vi "Reset Sensors.vi"   [LabVIEW 2014]
uses:
  Elevator/Elevator Control Command.ctl
  Elevator/Elevator Command.ctl
  Common Code/Elevator Mode.ctl
  Robot Global Data.vi
types:
  T1 = typedef "Elevator Command.ctl" = enum16{"Idle", "Load 1", "Load 2", "Load 3", "Drop Stack", "Eject Stack", "Untip Trashcan", "Load Trashcan"}
  T2 = typedef "Elevator Mode.ctl" = enum16{"Manual", "Safe", "Auto"}
  T3 = typedef "Elevator Control Command.ctl" = cluster{"Command":T1, "Manual Motor Out":dbl, "Manual Eject Piston":bool, "Mode":T2, "Override Limits":bool, "Manual Stabilizer":bool, "Manual Finger":bool, "Load from Step?":bool, "Store Trashcan?":bool, "Hold Low?":bool}
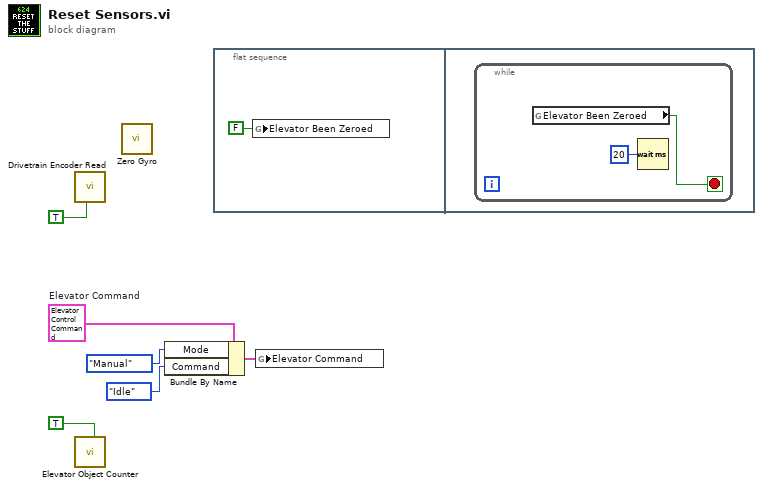
[diagram p0: block diagram]
diagram:
  w5 = T3 {"Command"=enum."Idle", "Manual Motor Out"=0.007874015748031496, "Manual Eject Piston"=FALSE, "Mode"=enum."Auto", "Override Limits"=FALSE, "Manual Stabilizer"=FALSE, "Manual Finger"=FALSE, "Load from Step?"=FALSE, "Store Trashcan?"=FALSE, "Hold Low?"=FALSE}  # Elevator Command
  n1 = call "Drivetrain Encoder Read.vi"("Reset?"=TRUE) -> ()  [unwired: 10 in, 1 out]
  n2 = call "Elevator Object Counter.vi"("Clear Stack?"=TRUE) -> ()  [unwired: 9 in, 2 out]
  n3 = call "Zero Gyro.vi"() -> ()  [unwired: 12 in]
  n4 = Bundle By Name(cluster=w5, "Mode"=Elevator_Mode."Manual", "Command"=Elevator_Command."Idle") -> (w4:T3)
  n5 = flat-sequence {
    frame #0 {
      n6 = global write "Robot Global Data.vi" "Elevator Been Zeroed"(FALSE ("Elevator Been Zeroed")) -> ()
    }
    frame #1 {
      n7 = while {
        stop <- w9 stop-if-true
        n8 = global read "Robot Global Data.vi" "Elevator Been Zeroed"() -> (w9:bool)
        n9 = Wait (ms)(milliseconds to wait=u32 20) -> ()  [unwired: 1 out]
      }
    }
  }
  n10 = global write "Robot Global Data.vi" "Elevator Command"(w4) -> ()
